vi "Go to Goal and Avoid Obstacle UM.vi"(0 "Robot Frame (World)":cluster{"X":sgl, "Y":sgl, "Theta":dbl}, 5 "Posture In":dbl[](array[numeric]), 7 "Goal Frame (World)":cluster{"X":sgl, "Y":sgl, "Theta":dbl}, 9 "IF readings\n(meters)":dbl[](array[numeric]) format="%_6g", 11 "V Forward":dbl=3.1) -> (4 "Frame Velocity":dbl[](array[numeric]))   [LabVIEW 2016]
uses:
  <vilib>/Analysis/coordinate.llb/Angle Units.ctl
  <vilib>/Analysis/coordinate.llb/Angle Range (Degree).ctl
  <vilib>/Analysis/baseanly.llb/Unit Vector (DBL).vi
  <vilib>/Analysis/coordinate.llb/Wrap Angle (scalar).vi
  <vilib>/Analysis/NI_AAL_Angle.lvlib
  <vilib>/Analysis/NI_AALBase.lvlib
panel:
  out "desired angle (rf)":dbl
  out "coerced(x)":dbl
  in  "Ratio Avoid and Goal":dbl=0.4
  out "Obs Vect (rf)":dbl[](array[numeric])
  out "Goal Vect (rf)":sgl[](array[numeric])
  in  "Sensor Gain":dbl[](array[numeric])=[1.0, 1.0, 0.5, 1.0, 1.0]
  out "ir distances wf":dbl[][](array[numeric])
  out "delta alpha":dbl
  in  "K":dbl=15.0
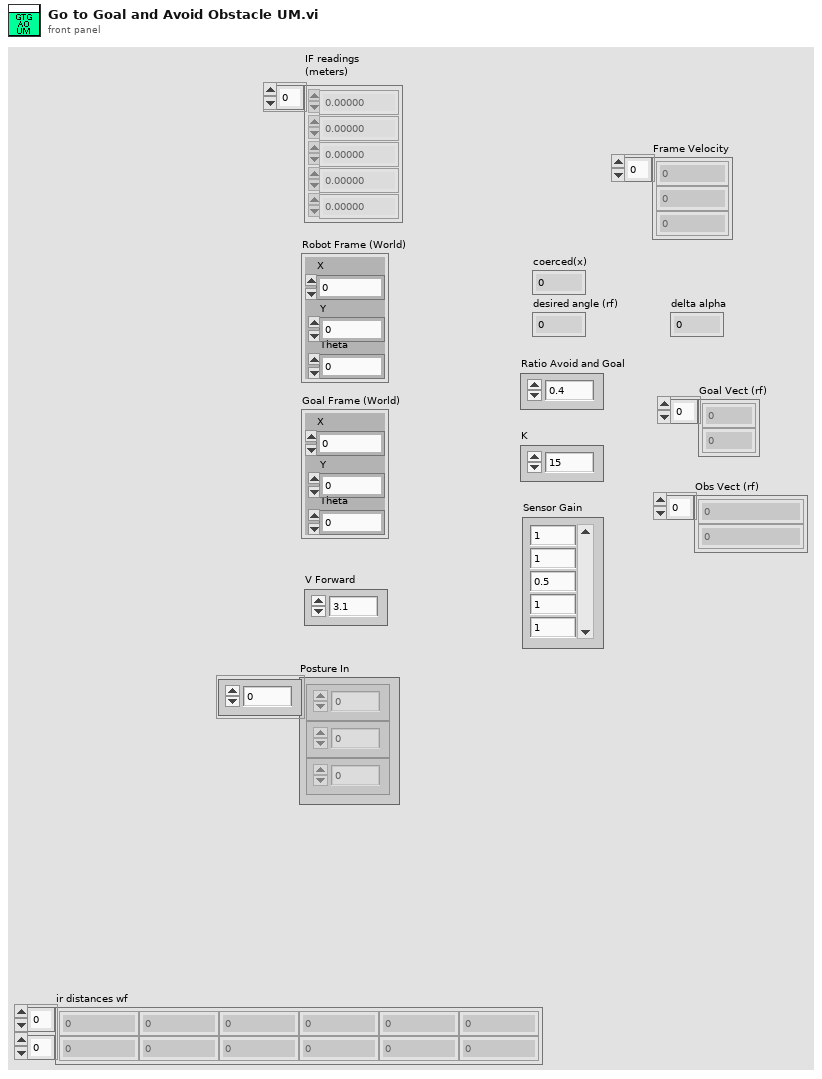
[diagram p1: front panel]
types:
  T1 = typedef "NI_AAL_Angle.lvlib/Angle Range (Degree).ctl" = u16
  T2 = typedef "NI_AAL_Angle.lvlib/Angle Units.ctl" = i32
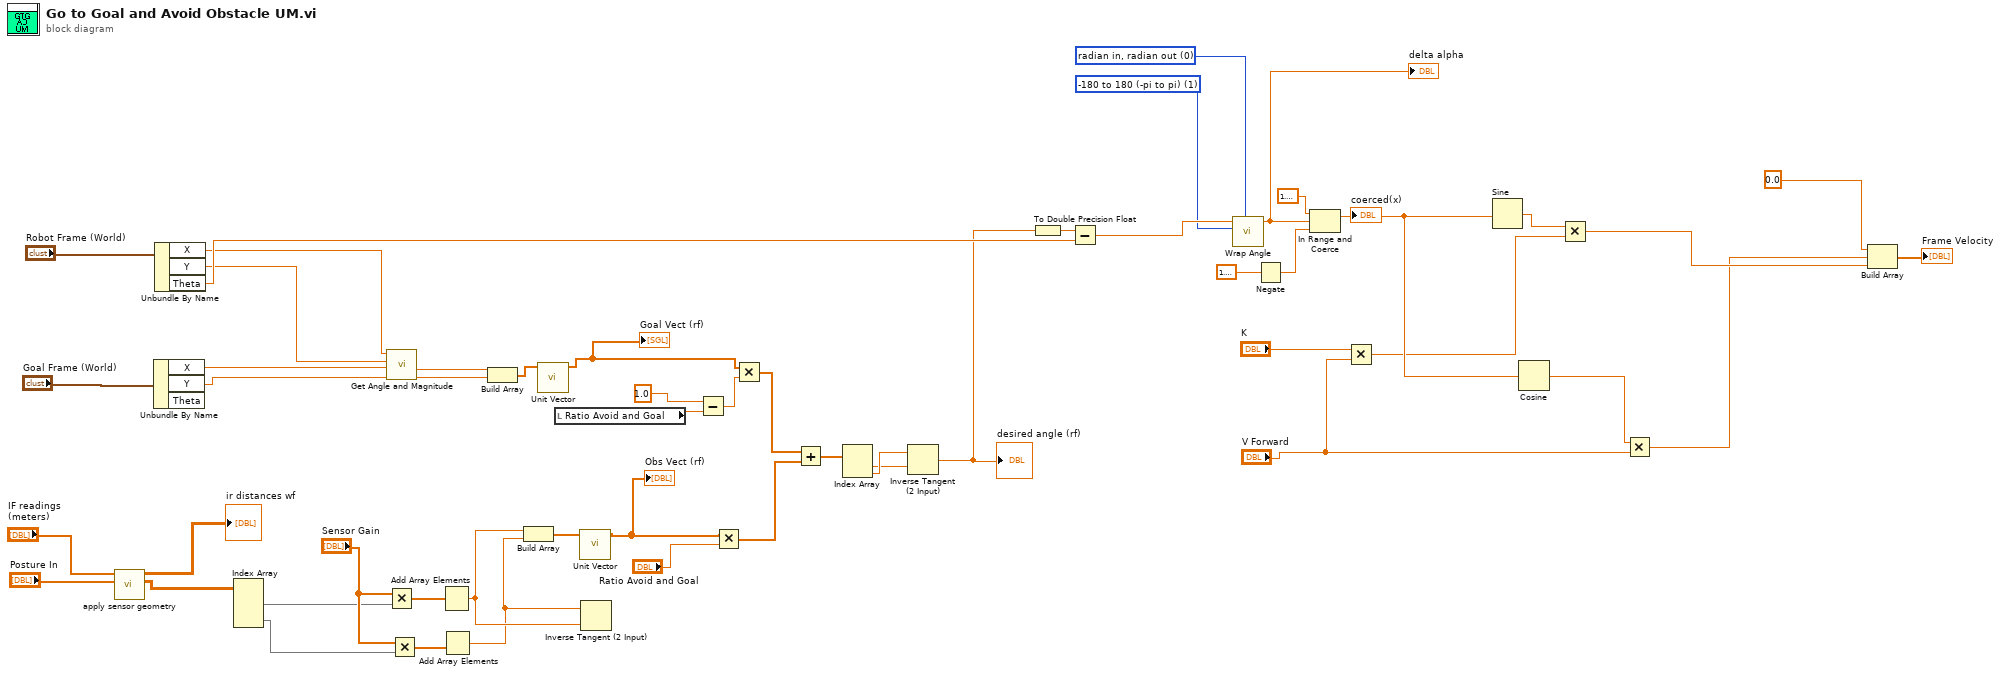
[diagram p0: block diagram]
diagram:
  w48 = T1 1 items=["none", "-180 to 180 (-pi to pi)", "0 to 360 (0 to 2pi)"] ("angle range")
  w49 = T2 0 items=["radian in, radian out", "radian in, degree out", "degree in, degree out", "degree in, radian out"] ("angle units")
  n1 = call "apply sensor geometry.vi"("Posture In"="Posture In", "IF readings\n(meters)"="IF readings\n(meters)") -> ("ir distances rf"=w38:dbl[][], "ir distances wf"=→"ir distances wf":dbl[][])  [unwired: 8 in]
  n2 = Unbundle By Name("Goal Frame (World)") -> ("X"=w33:sgl, "Y"=w32:sgl)  [unwired: 1 out]
  n3 = Unbundle By Name("Robot Frame (World)") -> ("X"=w35:sgl, "Y"=w34:sgl, "Theta"=w45:dbl)
  n4 = Index Array(array=w38) -> (element #1=w37:dbl[], element #2=w36:dbl[])  [unwired: 4 in]
  n5 = call "Get Angle and Magnitude.vi"("YGoal"=w32, "XGoal"=w33, "Y"=w34, "X"=w35) -> ("delta Y"=w29:sgl, "delta X"=w30:sgl)  [unwired: 4 in, 2 out]
  n6 = Multiply(x="Sensor Gain", y=w37) -> (x*y=w40:dbl[])
  n7 = Multiply(x="Sensor Gain", y=w36) -> (x*y=w39:dbl[])
  n8 = Add Array Elements(numeric array=w40) -> (sum=w28:dbl)
  n9 = Add Array Elements(numeric array=w39) -> (sum=w27:dbl)
  n10 = Build Array(w30, w29) -> (w4:sgl[])
  n11 = Build Array(w28, w27) -> (w2:dbl[])
  n12 = call-poly <vilib>:"Unit Vector.vi"("Input Vector"=w4) -> ("Unit Vector"=w3:dbl[])  [unwired: 8 in, 2 out]
  "Goal Vect (rf)" <- w3
  n13 = local read "Ratio Avoid and Goal"() -> (w25:dbl)
  n14 = call-poly <vilib>:"Unit Vector.vi"("Input Vector"=w2) -> ("Unit Vector"=w1:dbl[])  [unwired: 8 in, 2 out]
  "Obs Vect (rf)" <- w1
  n15 = Inverse Tangent (2 Input)(1:w28, 2:w27) -> ()  [unwired: 1 out]
  n16 = Subtract(x=1.0, y=w25) -> (x-y=w23:dbl)
  n17 = Multiply(x=w1, y="Ratio Avoid and Goal") -> (x*y=w21:dbl[])
  n18 = Multiply(x=w3, y=w23) -> (x*y=w22:dbl[])
  n19 = Add(x=w22, y=w21) -> (x+y=w20:dbl[])
  n20 = Index Array(array=w20) -> (element #1=w18:dbl, element #2=w19:dbl)  [unwired: 2 in]
  n21 = Inverse Tangent (2 Input)(1:w18, 2:w19) -> (0:w17:dbl)
  "desired angle (rf)" <- w17
  n22 = To Double Precision Float(number=w17) -> (double precision float=w31:dbl)
  n23 = Subtract(x=w31, y=w45) -> (x-y=w50:dbl)
  n24 = call-poly <vilib>:"Wrap Angle.vi"("angle units"=w49, "angle range"=w48, "angle in"=w50) -> ("angle out"=w14:dbl)  [unwired: 7 in, 1 out]
  "delta alpha" <- w14
  n25 = Negate(x=1.5707963267948966) -> (-x=w11:dbl)
  n26 = In Range and Coerce(upper limit=1.5707963267948966, x=w14, lower limit=w11) -> (coerced(x)=w10:dbl)  [unwired: 1 out]
  "coerced(x)" <- w10
  n27 = Multiply(x="K", y="V Forward") -> (x*y=w6:dbl)
  n28 = Sine(x=w10) -> (sin(x)=w16:dbl)
  n29 = Cosine(x=w10) -> (cos(x)=w9:dbl)
  n30 = Multiply(x=w16, y=w6) -> (x*y=w15:dbl)
  n31 = Multiply(x=w9, y="V Forward") -> (x*y=w8:dbl)
  n32 = Build Array(0.0 ("index"), w8, w15) -> (→"Frame Velocity":dbl[])
